vi "SpectrumAxis.vi"(9 "FFT Size":i32, 10 "SampleFreq":dbl, 11 "CarrierFreqz)":dbl) -> (2 "SpectrumConstant":cluster{"f0":dbl, "df":dbl, "magnitude":dbl[]})   [LabVIEW 2020]
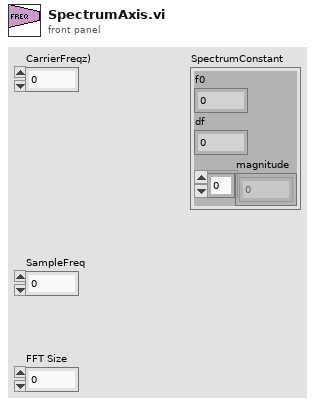
[diagram p1: front panel]
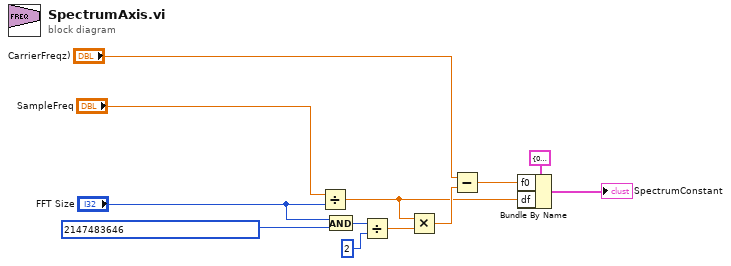
[diagram p0: block diagram]
diagram:
  n1 = Divide(x="SampleFreq", y="FFT Size") -> (x/y=w7:dbl)
  n2 = And(x="FFT Size", y=2147483646) -> (x .and. y?=w4:i32)
  n3 = Divide(x=w4, y=2) -> (x/y=w6:dbl)
  n4 = Multiply(x=w7, y=w6) -> (x*y=w9:dbl)
  n5 = Subtract(x="CarrierFreqz)", y=w9) -> (x-y=w8:dbl)
  n6 = Bundle By Name(cluster=cluster{"f0":dbl, "df":dbl, "magnitude":dbl[]} {"f0"=0.0, "df"=0.0, "magnitude"=[]} ("Power Spectrum / PSD"), "f0"=w8, "df"=w7) -> (→"SpectrumConstant":cluster{"f0":dbl, "df":dbl, "magnitude":dbl[]})
